vi "sudokufinal.vi"() -> ()   [LabVIEW 2023]
panel:
  out "M":string
  out "Cell rect":cluster{dbl, dbl, dbl, dbl}
  out "error out":errorcluster
  out "standard error Matlab":string
  out "standard output Matlab":string
  in  "Boolean":bool=TRUE
  out "standard error":string
  out "standard output":string
  out "1 - bit pixmap":bool[][](array[boolean])
  out "Hauteur":i16
  out "Largeur":i16
  out "BW picture":picture
  out "sudoku picture":picture
  in  "path to Jpeg file":path
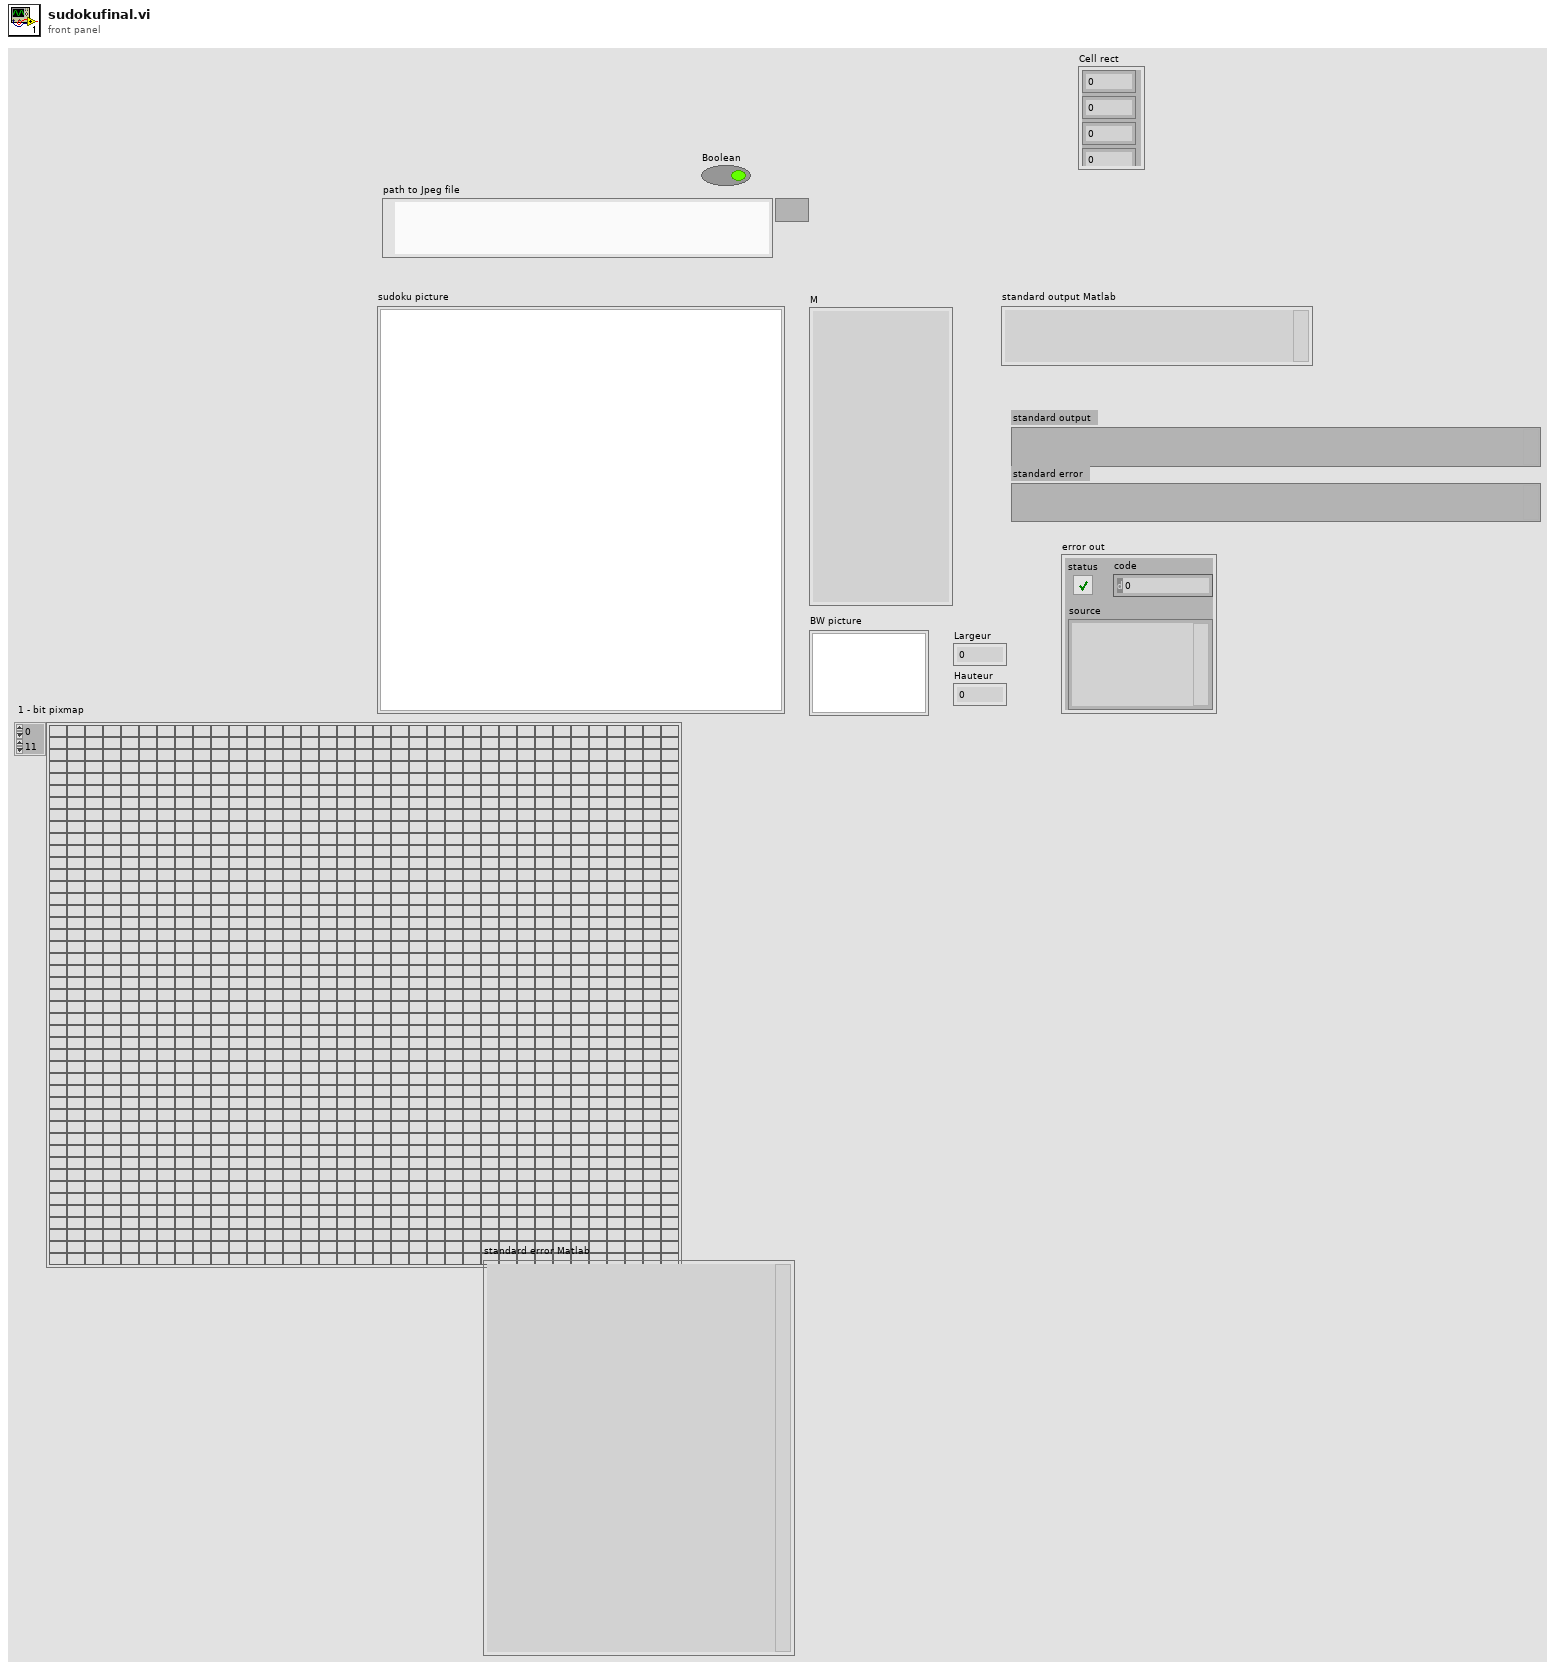
[diagram p1: front panel]
types:
  T1 = typedef "imagedata.ctl" = cluster{"image type":i32, "image depth":i32, "image":u8[], "mask":u8[], "colors":u32[], "Rectangle":cluster{"left":i16, "top":i16, "right":i16, "bottom":i16}}
  T2 = enum16{"open", "replace", "create", "open or create", "replace or create", "replace or create with confirmation"}
  T3 = enum16{"big-endian, network order", "native, host order", "little-endian"}
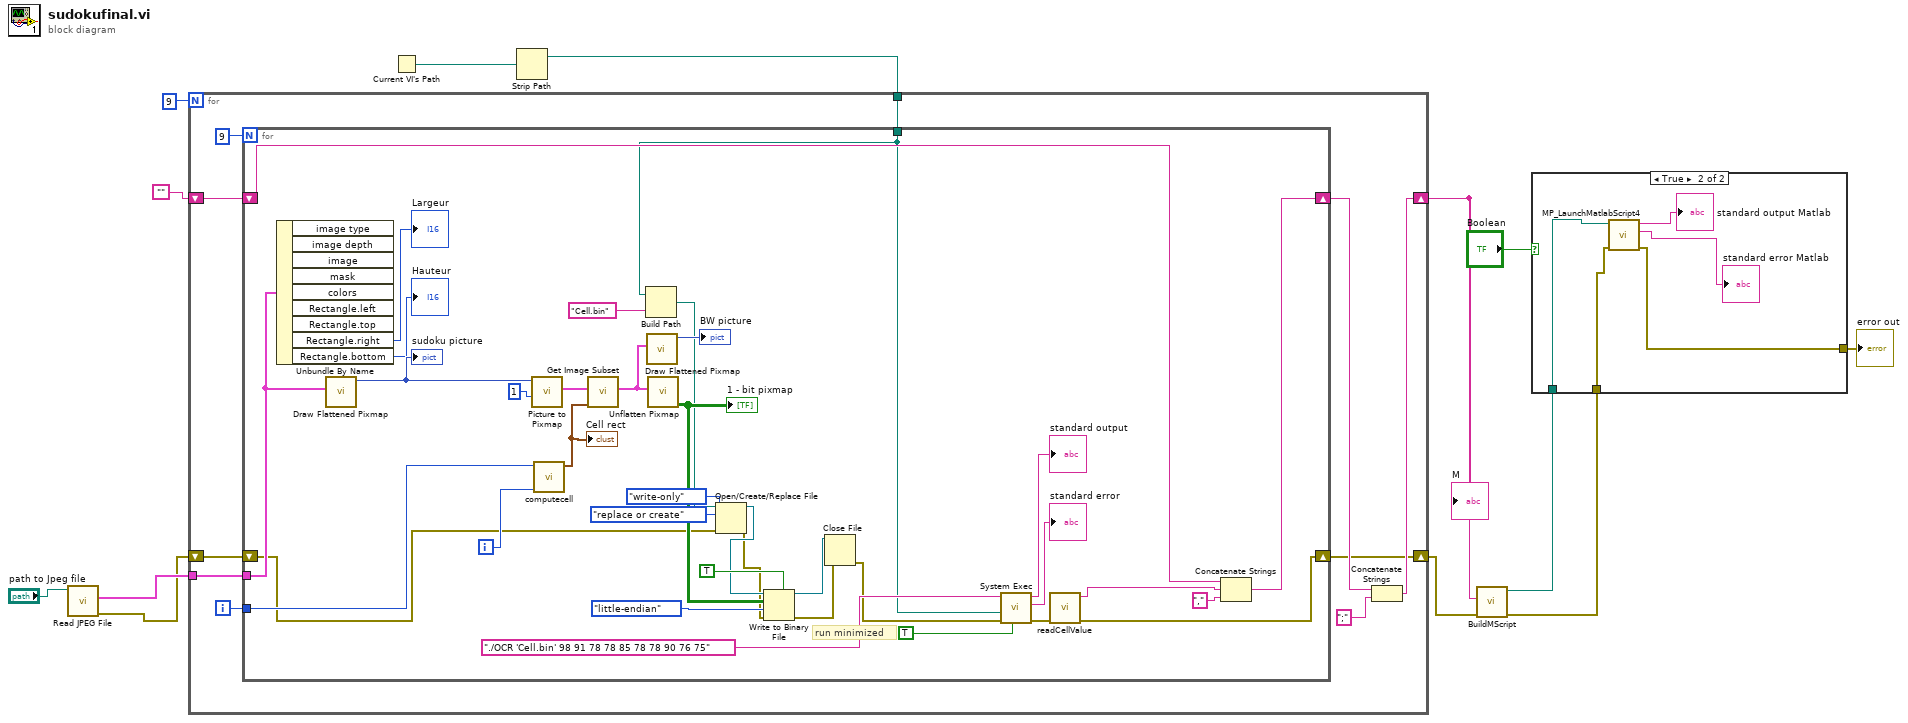
[diagram p0: block diagram]
diagram:
  n1 = call <vilib>:"Read JPEG File.vi"("path to JPEG file"="path to Jpeg file") -> ("error out"=w1:errorcluster, "image data"=w13:T1)  [unwired: 8 in, 1 out]
  n2 = Current VI's Path() -> (path=w4:path)
  n3 = Strip Path(path=w4) -> (stripped path=w5:path)  [unwired: 1 out]
  n4 = for {
    N: 9 -> [_]
    tunnel: w13 -> [w23]
    shift-right: [w19] -> w3
    shift-left: "" -> [w20]
    shift-right: [w16] -> w6
    shift-left: w1 -> [w14]
    tunnel: w5 -> [w15]
    i -> [w21]
    n5 = for {
      N: 9 -> [_]
      tunnel: w23 -> [w51]
      tunnel: w21 -> [w38]
      shift-right: [w41] -> w18
      shift-left: w20 -> [w42]
      shift-right: [w40] -> w16
      shift-left: w14 -> [w24]
      tunnel: w15 -> [w27]
      i -> [w36]
      # "run minimized"
      n6 = Unbundle By Name(w51) -> ("Rectangle.right"=→"Largeur":i16, "Rectangle.bottom"=→"Hauteur":i16)  [unwired: 7 out]
      n7 = call <vilib>:"Draw Flattened Pixmap.vi"("image data"=w51) -> ("new picture"=w57:picture)  [unwired: 8 in]
      "sudoku picture" <- w57
      n8 = call <vilib>:"Picture to Pixmap.vi"("depth"=1, "picture"=w57) -> ("image data"=w55:T1)  [unwired: 8 in, 1 out]
      n9 = call "computecell.vi"("i2"=w36, "i1"=w38) -> ("Cell rect"=w39:cluster{dbl, dbl, dbl, dbl})  [unwired: 9 in]
      "Cell rect" <- w39
      n10 = call <vilib>:"Get Image Subset.vi"("subset rect"=w39, "image data"=w55) -> ("image subset"=w54:T1)  [unwired: 4 in, 1 out]
      n11 = Build Path(base path=w27, name or relative path="Cell.bin") -> (appended path=w33:path)
      n12 = call <vilib>:"Draw Flattened Pixmap.vi"("image data"=w54) -> ("new picture"=→"BW picture":picture)  [unwired: 8 in]
      n13 = call <vilib>:"Unflatten Pixmap.vi"("image data"=w54) -> ("1-bit pixmap"=w50:bool[][])  [unwired: 4 in, 6 out]
      "1 - bit pixmap" <- w50
      n14 = Open/Create/Replace File(file path (use dialog)=w33, error in=w24, operation (0:open)=T2."replace or create", access (0:read/write)=enum16{"read/write", "read-only", "write-only"}."write-only") -> (refnum out=w32:refnum<file>, error out=w30:errorcluster)  [unwired: 2 in, 1 out]
      n15 = Write to Binary File(file (use dialog)=w32, data=w50, error in=w30, 5:TRUE, 9:T3."little-endian" ("byte order (0:big-endian, network order)")) -> (refnum out=w31:refnum<file>, error out=w29:errorcluster)  [unwired: 1 in, 1 out]
      n16 = Close File(refnum=w31, error in=w29) -> (error out=w28:errorcluster)  [unwired: 1 out]
      n17 = call <vilib>:"System Exec.vi"("run minimized? (F)"=TRUE ("run minimized"), "error in (no error)"=w28, "working directory"=w27, "command line"="./OCR 'Cell.bin' 98 91 78 78 85 78 78 90 76 75") -> ("error out"=w44:errorcluster, "standard error"=→"standard error":string, "standard output"=→"standard output":string)  [unwired: 4 in, 1 out]
      n18 = call "readCellValue.vi"("error in (no error)"=w44) -> ("error out"=w40:errorcluster, "resulting string"=w37:string)  [unwired: 9 in]
      n19 = Concatenate Strings(w42, w37, "," ("string")) -> (w41:string)
    }
    n20 = Concatenate Strings(w18, ";" ("string")) -> (w19:string)
  }
  "M" <- w3
  n21 = call "BuildMScript.vi"("error in"=w6, "string"=w3) -> ("error out"=w9:errorcluster, "appended path"=w7:path)  [unwired: 8 in]
  n22 = case shown="True" "Boolean" {
    tunnel: w9 -> [w59 w62]
    tunnel: [w59 w61] -> w8
    tunnel: w7 -> [_ w60]
    frame False {
    }
    frame True {
      n23 = call "MP_LaunchMatlabScript4.vi"("error in (no error)"=w62, "matlab script path"=w60) -> ("error out"=w61:errorcluster, "standard error"=→"standard error Matlab":string, "standard output"=→"standard output Matlab":string)  [unwired: 4 in, 3 out]
    }
  }
  "error out" <- w8
